vi "LabVIEW FPGA FFT_v2.vi"() -> ()   [LabVIEW 2020]
doc: "This FPGA VI illustrates use of the FFT in a single-cycle Timed Loop (SCTL). The FFT returns results in a \"burst\" fashion, requiring several calls on average for each valid output result.\n\nThe entire data pipeline uses a handshaking protocol to ensure that no data is lost, by throttling upstream nodes if any node is not ready to receive data. If the pipeline is too slow (as determined by the host VI DMA Read loop), the Sine Wave FIFO will eventually overflow, returning Timed Out? and notifies the host UI."
uses:
  Type Definitions/Windows.ctl
  <vilib>/Platform/TimedLoop/XDataNode/timing_clust.ctl
  <vilib>/Platform/TimedLoop/XDataNode/nitl_modes.ctl
  <vilib>/Platform/TimedLoop/XDataNode/wakeup.ctl
  <vilib>/rvi/Analysis/measure/FFT/simModelSupport/niFPGA FFT Sim Properties.ctl
  <vilib>/rvi/Analysis/measure/FFT/simModelSupport/niFPGA FFT Sim Types.ctl
  <vilib>/rvi/Analysis/measure/FFT/simModelSupport/niFpgaFFTSimArithmeticProperties.ctl
  <vilib>/rvi/Analysis/measure/FFT/simModelSupport/niFpgaFFTSimDfxp.ctl
  <vilib>/fxp/LVFixedPointQuantizationPolicyTypeDef.ctl
  <vilib>/rvi/eio/common/nirviEmuTemplateMethod_errors.vi
  <vilib>/rvi/Emulation/niFpgaGetClockAttributes.vi
  <vilib>/rvi/Emulation/niFpgaSctlEmulationGetInTimedLoop.vi
  <vilib>/rvi/Emulation/niFpgaEmulationReportErrorSimple.vi
  <vilib>/rvi/DataTransferAndStorage/Container/Common/niFpgaContainerGetUniqueNameForEmu.vi
  <vilib>/rvi/DataTransferAndStorage/Container/Common/niFpgaContainerSetEmuInfo.vi
  <vilib>/rvi/eio/common/nirviEmuReportErrorAndStop.vi
  <vilib>/rvi/Emulation/niFpgaCriticalErrorInLSC.vi
  <vilib>/rvi/interface/RandomDataEmulation/niFpgaRandomDataHandleErrors.vi
  <vilib>/rvi/DataTransferAndStorage/Container/Common/niFpgaContainerExecOnDevCompGetState.vi
  <vilib>/rvi/Emulation/niFpgaEmulationIsFPGAContextNoSignature.vi
  <vilib>/rvi/errors/niFpgaSetErrorForExecOnDevCompSimple.vi
  <vilib>/rvi/FIFO/Fifo_Resource/nirvififoEmulationSetSize.vi
  <vilib>/rvi/FIFO/Fifo_Resource/nirviFifoEmulationQueueMgr.vi
  <instcachedir>/0/nirviFifoEmulationQueueMgr_E5CAEC123FF24DC58D834DCA3CDAA9B5.lvgen/nirviFifoEmulationQueueMgr_E5CAEC123FF24DC58D834DCA3CDAA9B5_002.vi
  <vilib>/rvi/FIFO/Fifo_Resource/nirvififoEmulationDetermineInputValidOut.vi
  <vilib>/rvi/FIFO/Fifo_Resource/nirvififoEmulationCreateLock.vi
  <vilib>/rvi/Emulation/niFpgaProcessEmulError.vi
  <vilib>/rvi/FIFO/Fifo_Resource/nirvififoEmulationObtainLock.vi
  <vilib>/rvi/FIFO/Fifo_Resource/nirvififoEmulationReleaseLock.vi
  <vilib>/rvi/occurrence/nirviWaitOnOccurrenceBase.vi
  <vilib>/rvi/errors/nirviReportUnexpectedCaseInternalError.vi
  <vilib>/rvi/errors/nirviReportUnexpectedCaseInternalError (U32).vi
  <vilib>/Utility/error.llb/Clear Errors.vi
  <vilib>/rvi/Analysis/measure/FFT/simModelSupport/niFpgaFFTSimModelCore.vi
  <vilib>/eio/EIONode/EIONode.xnode
  <vilib>/Platform/TimedLoop/XDataNode/XDataNode.xnode
  <vilib>/rvi/LocalResourceManager/LocalResourceManager.xnode
  <vilib>/rvi/DataTransferAndStorage/Container/XNode/niFpgaContainer.xnode
  <vilib>/rvi/interface/RandomDataEmulation/nirviRandomDataFpgaReadWriteTemplate.vi
  <vilib>/rvi/FIFO/Fifo_Resource/niFpgaFifoEmulationRefIn.vi
  <vilib>/rvi/Analysis/measure/FFT/XNode/niFpgaFFT.xnode
  <vilib>/Platform/TimedLoop/XDataNode/XDNodeRunTimeDep.lvlib
panel:
  in  "Window select":T1=enum."None"
  out "Overflow":bool
  out "Actual Sample Period (ticks)":u32
  in  "Frequency (periods/tick)":fxp<+,32,0>=0.0002500000409781933
  out "Invalid Period":bool
  in  "Requested Sample Period (ticks)":u32=1000
  # "Overview: Demonstrates the use of the LabVIEW FPGA FFT function for custom in-hardware signal processing\nRequirements: LabVIEW FPGA Module, NI-RIO\nInstructions: Run the VI"
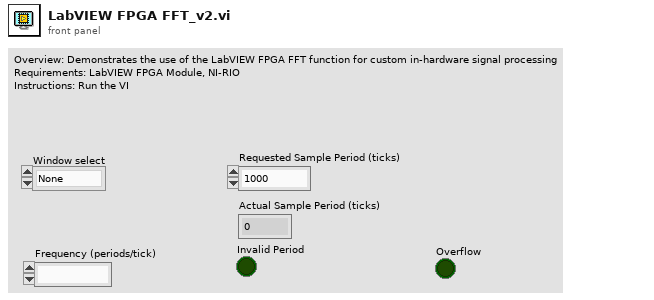
[diagram p1: front panel]
types:
  T1 = typedef "Windows.ctl" = enum16{"Hamming", "Hanning", "None"}
  T2 = typedef "XDNodeRunTimeDep.lvlib/timing_clust.ctl" = cluster{"Expected End [f-1]":u64, "Actual End [f-1]":u64, "Finished Late? [f-1]":bool, "Expected End [i-1]":u64, "Actual End [i-1]":u64, "Finished Late? [i-1]":bool, "Expected Start [i]":u64, "Actual Start [i]":u64, "Expected Start [f]":u64, "Actual Start [f]":u64, "Source Name":string, "Structure Name":string, "Period":i64, "Deadline":i64, "Offset":i64, "Start":i64, "Priority":i32, "Timeout":i32, "Mode":T3, "Wakeup Reason":T4, "Error":errorcluster, "Source Type":string, "Secondary Source Type":string, "Global End Time":u64, "Global Start Time":u64, "Frame Duration":u64, "Iteration Duration":u64, "Assigned CPU":i32, "I/O Scan Engine Mode":u32}
  T3 = typedef "XDNodeRunTimeDep.lvlib/nitl_modes.ctl" = enum32{"No Change", "Process missed periods, maintain original phase", "Discard missed periods, maintain original phase", "Process missed periods, ignore original phase", "Discard missed periods, ignore original phase"}
  T4 = typedef "XDNodeRunTimeDep.lvlib/wakeup.ctl" = enum32{"Normal", "Aborted", "Asynchronous wakeup", "Timing source error", "Timed loop error", "Timeout"}
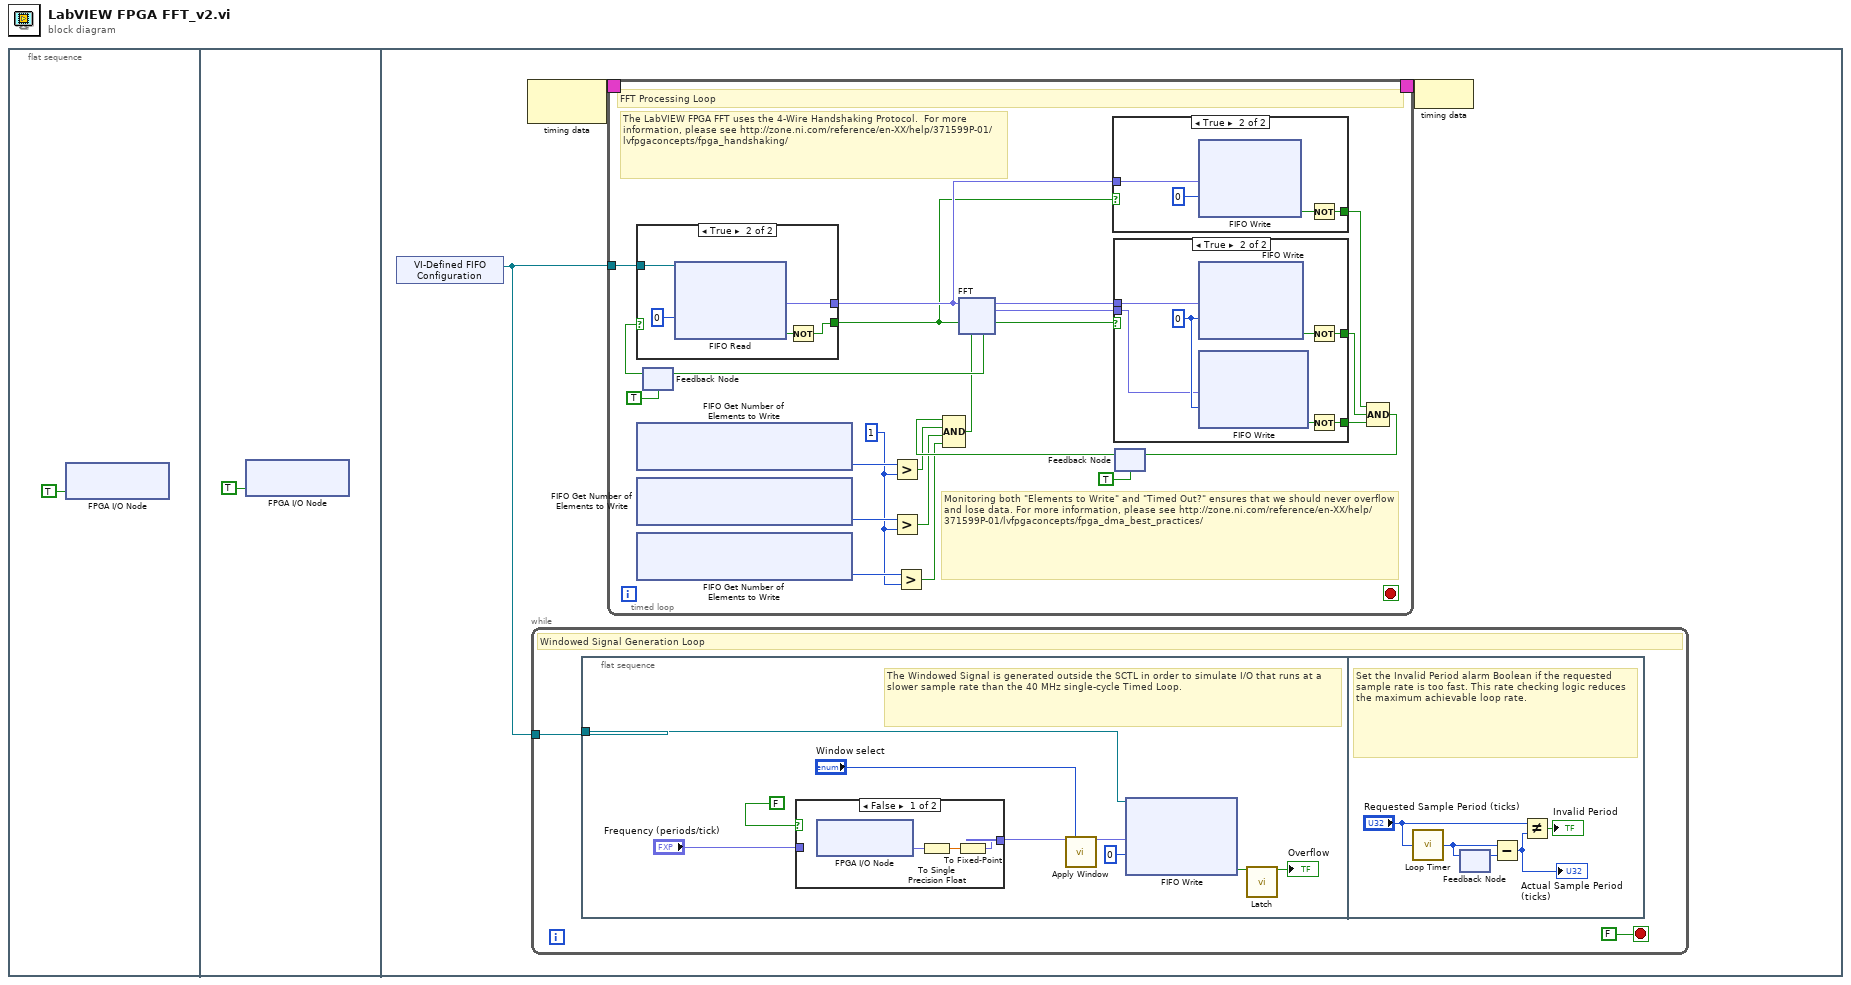
[diagram p0: block diagram]
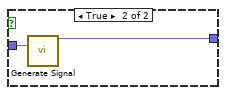
[diagram p2: hidden frame]
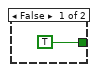
[diagram p3: hidden frame]
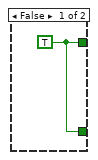
[diagram p4: hidden frame]
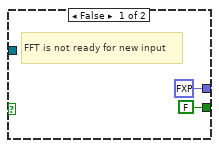
[diagram p5: hidden frame]
diagram:
  n1 = flat-sequence {
    frame #0 {
      n2 = xnode "FPGA I/O Node"("Mod1/Stop"=TRUE) -> ()  [unwired: 1 in, 1 out]
    }
    frame #1 {
      n3 = xnode "FPGA I/O Node"("Mod1/Start"=TRUE ("Mod1/Stop")) -> ()  [unwired: 1 in, 1 out]
    }
    frame #2 {
      n4 = xnode "VI-Defined FIFO Configuration"() -> ("FIFO Out"=w3:refnum<k21>)
      n5 = node-c288() -> (w5:T2)  [unwired: 1 in]
      n6 = while {
        tunnel: w3 -> [w7]
        stop <- FALSE stop-if-true
        # "Windowed Signal Generation Loop"
        n7 = flat-sequence {
          tunnel: w7 -> [w12]
          frame #0 {
            # "The Windowed Signal is generated outside the SCTL in order to simulate I/O that runs at a slower sample rate than the 40 MHz single-cycle Timed Loop."
            n8 = case shown="False" FALSE {
              tunnel: [w17 w21] -> w13
              tunnel: "Frequency (periods/tick)" -> [_ w20]
              frame False {
                n9 = xnode "FPGA I/O Node"() -> ("Mod1/AI0"=w19:fxp<+/-,24,7>)  [unwired: 1 in, 1 out]
                n10 = To Single Precision Float(number=w19) -> (single precision float=w18:sgl)
                n11 = To Fixed-Point(number=w18) -> (fixed-point=w17:fxp<+/-,16,5>)  [unwired: 1 in]
              }
              frame True {
                n12 = call "Generate Signal.vi"("frequency (periods/tick)"=w20) -> ("signal"=w21:fxp<+/-,16,5>)  [unwired: 14 in]
              }
            }
            n13 = call "Apply Window.vi"("Signal In"=w13, "Window select"="Window select") -> ("Windowed Signal Out"=w14:fxp<+/-,16,5>)  [unwired: 13 in]
            n14 = xnode ("FIFO Write")("Element"=w14, "Timeout"=0, "FIFO In"=w12) -> ("Timed Out?"=w11:bool)  [unwired: 1 out]
            n15 = call "Latch.vi"("Input"=w11) -> ("Output"=→"Overflow":bool)  [unwired: 14 in]
          }
          frame #1 {
            # "Set the Invalid Period alarm Boolean if the requested sample rate is too fast. This rate checking logic reduces the maximum achievable loop rate."
            n16 = call "Loop Timer"("Count(Ticks)"="Requested Sample Period (ticks)") -> ("Tick Count(Ticks)"=w22:u32)
            n17 = feedback #1() -> (w23:u32)  [unwired: 1 in]
            n18 = feedback-in #1(w22) -> ()
            n19 = Subtract(x=w22, y=w23) -> (x-y=w26:u32)
            "Actual Sample Period (ticks)" <- w26
            n20 = Not Equal?(x="Requested Sample Period (ticks)", y=w26) -> (x != y?=→"Invalid Period":bool)
          }
        }
      }
      n21 = timed-loop {
        timing: w5 -> [_]
        timing-out: [_] -> w4
        tunnel: w3 -> [w45]
        stop <- _ stop-if-true
        w33 = u32 1 ("y")
        # "Monitoring both \"Elements to Write\" and \"Timed Out?\" ensures that we should never overflow and lose data. For more information, please see http://zone.ni.com/reference/en-XX/help/371599P-01/lvfpgaconcepts/fpga_dma_best_practices/"
        # "The LabVIEW FPGA FFT uses the 4-Wire Handshaking Protocol.  For more information, please see http://zone.ni.com/reference/en-XX/help/371599P-01/lvfpgaconcepts/fpga_handshaking/"
        # "FFT Processing Loop"
        n22 = xnode ("FIFO Get Number of Elements to Write")() -> ("Number of Elements to Write"=w36:u32)  [unwired: 1 in, 1 out]
        n23 = xnode ("FIFO Get Number of Elements to Write")() -> ("Number of Elements to Write"=w35:u32)  [unwired: 1 in, 1 out]
        n24 = xnode ("FIFO Get Number of Elements to Write")() -> ("Number of Elements to Write"=w34:u32)  [unwired: 1 in, 1 out]
        n25 = feedback #2(TRUE ("ready for input")) -> (w49:bool)
        n26 = case shown="True" w49 {
          tunnel: [FALSE w94] -> w46
          tunnel: [fxp<+/-,16,5> 0.0 ("Element") w95] -> w48
          tunnel: w45 -> [_ w91]
          frame False {
            # "FFT is not ready for new input"
          }
          frame True {
            n27 = xnode ("FIFO Read")("Timeout"=0, "FIFO In"=w91) -> ("Element"=w95:fxp<+/-,16,5>, "Timed Out?"=w93:bool)  [unwired: 1 out]
            n28 = Not(x=w93) -> (.not. x?=w94:bool)
          }
        }
        n29 = Greater?(x=w36, y=w33) -> (0:w30:bool)
        n30 = Greater?(x=w35, y=w33) -> (0:w29:bool)
        n31 = Greater?(x=w34, y=w33) -> (0:w28:bool)
        n32 = case shown="True" w46 {
          tunnel: w48 -> [_ w77]
          tunnel: [TRUE ("Timed Out?") w78] -> w41
          frame False {
          }
          frame True {
            n33 = xnode ("FIFO Write")("Element"=w77, "Timeout"=0) -> ("Timed Out?"=w79:bool)  [unwired: 1 in, 1 out]
            n34 = Not(x=w79) -> (.not. x?=w78:bool)
          }
        }
        n35 = feedback #3(TRUE) -> (w31:bool)
        n36 = Compound Arithmetic op=AND(w31, w30, w29, w28) -> (w32:bool)
        n37 = xnode "FFT"("real data in"=w48, "input valid"=w46, "ready for output"=w32) -> ("ready for input"=w47:bool, "real data out"=w44:fxp<+/-,26,15>, "imaginary data out"=w43:fxp<+/-,26,15>, "output valid"=w42:bool)  [unwired: 2 in, 1 out]
        n38 = feedback-in #2(w47) -> ()
        n39 = case shown="True" w42 {
          tunnel: w44 -> [_ w83]
          tunnel: w43 -> [_ w82]
          tunnel: [w81 w85] -> w40
          tunnel: [w81 w84] -> w39
          frame False {
            w81 = TRUE ("Timed Out?")
          }
          frame True {
            w88 = 0 ("Timeout")
            n40 = xnode ("FIFO Write")("Element"=w83, "Timeout"=w88) -> ("Timed Out?"=w87:bool)  [unwired: 1 in, 1 out]
            n41 = xnode ("FIFO Write")("Element"=w82, "Timeout"=w88) -> ("Timed Out?"=w86:bool)  [unwired: 1 in, 1 out]
            n42 = Not(x=w87) -> (.not. x?=w85:bool)
            n43 = Not(x=w86) -> (.not. x?=w84:bool)
          }
        }
        n44 = Compound Arithmetic op=AND(w41, w40, w39) -> (w38:bool)
        n45 = feedback-in #3(w38) -> ()
      }
      n46 = node-c288(w4) -> ()
    }
  }
